vi "JV Measurement_IIT.vi"(9 "Max (V)":dbl=1.4, 11 "Step (V)":dbl=0.01) -> ()   [LabVIEW 2011]
uses:
  <instrlib>/keithley_24xx/Keithley 24XX/Keithley 24XX.lvlib
panel:
  in  "Exit Program":bool
  in  "Boolean":bool
  in  "Device Structure":bool
  out "Log Table":string[][](table)
  out "JV Curve":cluster{"Y":dbl[], "Y":dbl[]}[](graph)
  in  "Initial scan direction":bool=TRUE
  in  "Measurement Delay (ms)":dbl=1.0
  in  "Sample Name":string
  in  "Device Area (cm^2)":dbl=0.12
  in  "Experiment Title":string
  in  "User Name":string
  in  "Stabilisation level \n(A or V depending on mode)":dbl=1.4
  in  "Stabilisation time (s)":dbl=5.0
  in  "Stabilisation mode":enum16{"Voltage", "Current"}(ring)
  in  "Min (V)":dbl
  # "Jsc"
  # "Voc"
  # "PCE"
  # "FF"
  # "Area"
  # "Sta. Lev."
  # "Sta. Time"
  # "Delay"
  # "File Path"
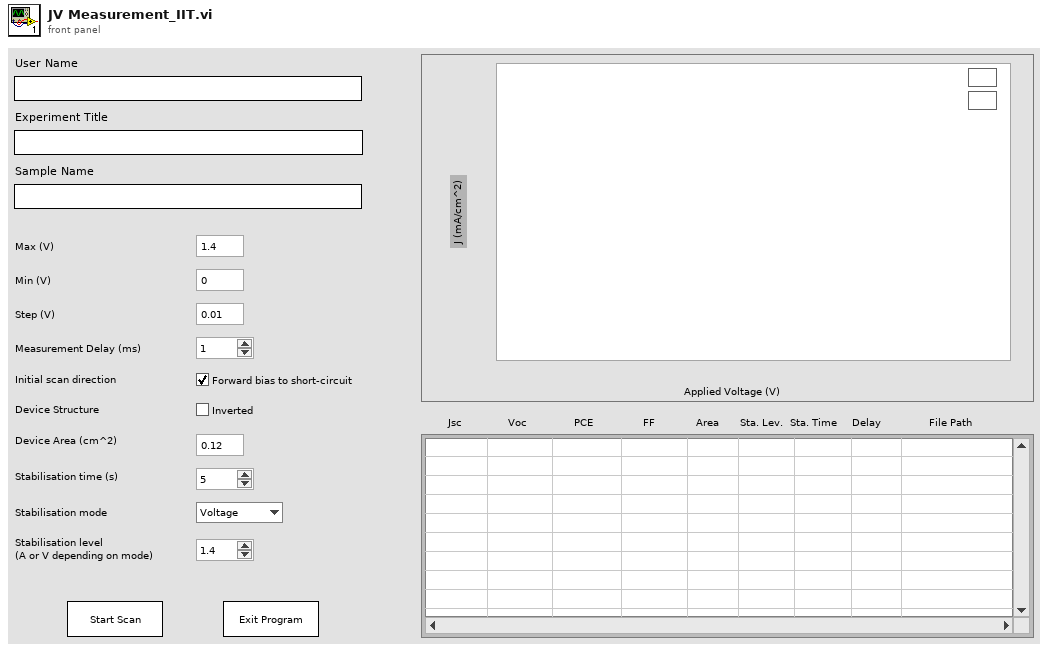
[diagram p1: front panel]
types:
  T1 = typedef "imagedata.ctl" = cluster{"image type":i32, "image depth":i32, "image":u8[], "mask":u8[], "colors":u32[], "Rectangle":cluster{"left":i16, "top":i16, "right":i16, "bottom":i16}}
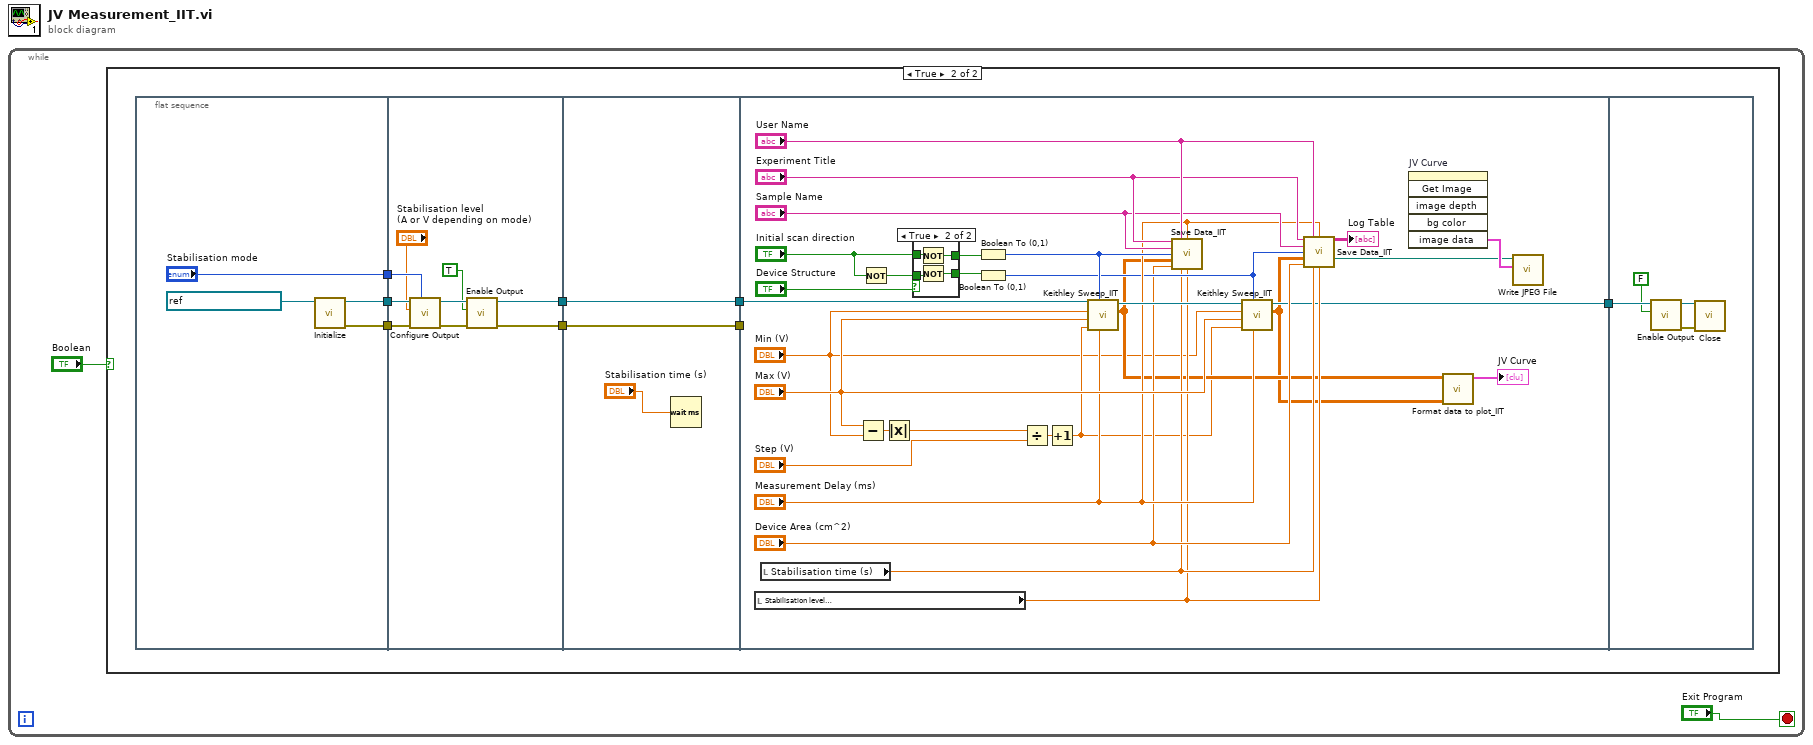
[diagram p0: block diagram]
diagram:
  n1 = while {
    stop <- "Exit Program" stop-if-true
    n2 = case shown="True" "Boolean" {
      frame False {
      }
      frame True {
        n3 = flat-sequence {
          tunnel: ["Stabilisation mode"] -> w10
          tunnel: [w11] -> w9
          tunnel: [w12] -> w8
          tunnel: w10 -> [w17]
          tunnel: w9 -> [w20]
          tunnel: w8 -> [w21]
          tunnel: [w19] -> w7
          tunnel: [w18] -> w6
          tunnel: [w26] -> w5
          tunnel: w7 -> [w26]
          tunnel: [w25] -> w4
          tunnel: w6 -> [w25]
          tunnel: w5 -> [w56]
          tunnel: w4 -> [_]
          tunnel: [w38] -> w3
          tunnel: w3 -> [w66]
          frame #0 {
            n4 = call <instrlib>:"Initialize.vi"("VISA resource name"=refnum<visa-resource-name> "GPIB0::24::INSTR") -> ("error out"=w11:errorcluster, "VISA resource name out"=w12:refnum<visa-resource-name>)  [unwired: 4 in, 5 out]
          }
          frame #1 {
            n5 = call <instrlib>:"Configure Output.vi"("Source Mode  (0: Voltage)"=w17, "error in (no error)"=w20, "Output Level (0)"="Stabilisation level \n(A or V depending on mode)", "VISA resource name"=w21) -> ("error out"=w23:errorcluster, "VISA resource name out"=w22:refnum<visa-resource-name>)  [unwired: 6 in]
            n6 = call <instrlib>:"Enable Output.vi"("error in (no error)"=w23, "Enable Output (T: Enable)"=TRUE ("Output (Off)"), "VISA resource name"=w22) -> ("error out"=w18:errorcluster, "VISA resource name out"=w19:refnum<visa-resource-name>)  [unwired: 7 in]
          }
          frame #2 {
            n7 = Wait (ms)(milliseconds to wait="Stabilisation time (s)") -> ()  [unwired: 1 out]
          }
          frame #3 {
            n8 = local read "Stabilisation level \n(A or V depending on mode)"() -> (w39:dbl)
            n9 = local read "Stabilisation time (s)"() -> (w40:dbl)
            n10 = Subtract(x="Max (V)", y="Min (V)") -> (x-y=w53:dbl)
            n11 = Not(x="Initial scan direction") -> (.not. x?=w29:bool)
            n12 = Absolute Value(x=w53) -> (abs(x)=w54:dbl)
            n13 = case shown="True" "Device Structure" {
              tunnel: [w58 w62] -> w31
              tunnel: [w57 w61] -> w30
              tunnel: w29 -> [w57 w60]
              tunnel: "Initial scan direction" -> [w58 w59]
              frame False {
              }
              frame True {
                n14 = Not(x=w59) -> (.not. x?=w62:bool)
                n15 = Not(x=w60) -> (.not. x?=w61:bool)
              }
            }
            n16 = Boolean To (0,1)(Boolean=w31) -> (0, 1=w49:i16)
            n17 = Boolean To (0,1)(Boolean=w30) -> (0, 1=w42:i16)
            n18 = Divide(x=w54, y="Step (V)") -> (x/y=w34:dbl)
            n19 = Increment(x=w34) -> (x+1=w33:dbl)
            n20 = call "Keithley Sweep_IIT.vi"("Source Delay (s)"="Measurement Delay (ms)", "Sweep Direction"=w49, "Number of Points"=w33, "Maximum Amplitude"="Max (V)", "Minimum Amplitude"="Min (V)", "VISA resource name out 2"=w56) -> ("Data Array"=w37:dbl[][], "VISA resource name out"=w48:refnum<visa-resource-name>)  [unwired: 1 in, 1 out]
            n21 = call "Save Data_IIT.vi"("Experiment Indicator"="Experiment Title", "Username"="User Name", "Measurement Delay (ms)"="Measurement Delay (ms)", "Sample Name"="Sample Name", "Scan direction"=w49, "Data Array"=w37, "Device Area (cm^2)"="Device Area (cm^2)", "Stabilisation time (ms)"=w40, "Stabilisation level \n(A or V depending on mode)"=w39) -> ()  [unwired: 3 in, 4 out]
            n22 = call "Keithley Sweep_IIT.vi"("Source Delay (s)"="Measurement Delay (ms)", "Sweep Direction"=w42, "Number of Points"=w33, "Maximum Amplitude"="Max (V)", "Minimum Amplitude"="Min (V)", "VISA resource name out 2"=w48) -> ("Data Array"=w36:dbl[][], "VISA resource name out"=w38:refnum<visa-resource-name>)  [unwired: 1 in, 1 out]
            n23 = call "Save Data_IIT.vi"("Experiment Indicator"="Experiment Title", "Username"="User Name", "Measurement Delay (ms)"="Measurement Delay (ms)", "Sample Name"="Sample Name", "Scan direction"=w42, "Data Array"=w36, "Device Area (cm^2)"="Device Area (cm^2)", "Stabilisation time (ms)"=w40, "Stabilisation level \n(A or V depending on mode)"=w39) -> ("Master Log"=→"Log Table":string[][], "File path for JV image"=w51:path)  [unwired: 3 in, 2 out]
            n24 = invoke on="JV Curve" class="XYGraph (strict)" method="Get Image"() -> ("image data"=w52:T1)  [unwired: 6 in, 5 out]
            n25 = call "Format data to plot_IIT.vi"("Data Array 2"=w36, "Data Array"=w37) -> ("JV Curve"=→"JV Curve":cluster{"Y":dbl[], "Y":dbl[]}[])  [unwired: 9 in]
            n26 = call <vilib>:"Write JPEG File.vi"("image data"=w52, "path to JPEG file"=w51) -> ()  [unwired: 8 in, 2 out]
          }
          frame #4 {
            n27 = call <instrlib>:"Enable Output.vi"("Enable Output (T: Enable)"=FALSE ("Output (Off)"), "VISA resource name"=w66) -> ("error out"=w64:errorcluster, "VISA resource name out"=w65:refnum<visa-resource-name>)  [unwired: 8 in]
            n28 = call <instrlib>:"Close.vi"("error in (no error)"=w64, "VISA resource name"=w65) -> ()  [unwired: 9 in, 1 out]
          }
        }
      }
    }
  }
